vi "Write Data Reference.vi"(8 "error in (no error)":errorcluster, 10 "Data Reference":refnum<data-value>, 11 "Abs_Waveform in":refnum<class "Abs_Waveform.lvclass">) -> (0 "error out":errorcluster, 3 "Abs_Waveform out":refnum<class "Abs_Waveform.lvclass">)   [LabVIEW 2021, in "Abs_Waveform.lvclass"]
uses:
  Abs_Waveform.lvclass
  Abs_Waveform.lvclass/Abs_Waveform.ctl
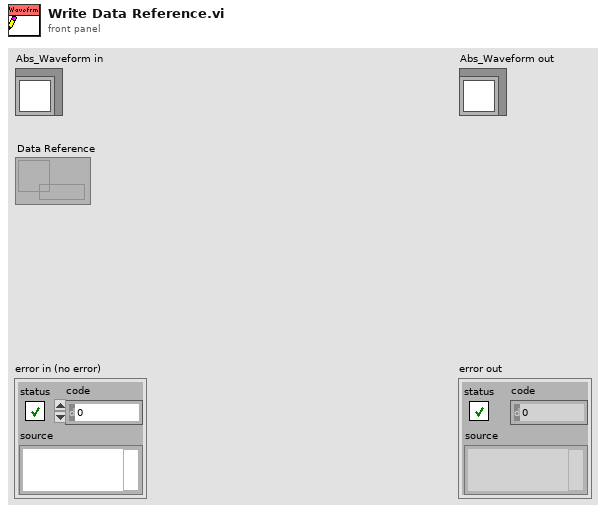
[diagram p1: front panel]
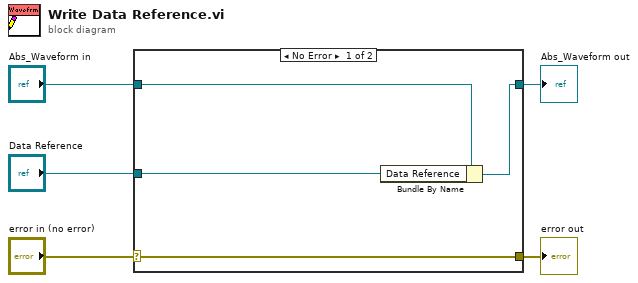
[diagram p0: block diagram]
diagram:
  n1 = case shown="No Error" "error in (no error)" {
    selector: "error in (no error)" -> [w9 w10]
    tunnel: [w9 w10] -> w4
    tunnel: [w7 w11] -> w2
    tunnel: "Abs_Waveform in" -> [w8 w11]
    tunnel: "Data Reference" -> [w6 _]
    frame No Error {
      n2 = Bundle By Name(cluster=w8, "Data Reference"=w6) -> (w7:refnum<class "Abs_Waveform.lvclass">)
    }
    frame Error {
    }
  }
  "error out" <- w4
  "Abs_Waveform out" <- w2
